vi "New_camera_Configuration_testcode.vi"(5 "Exposure time":dbl, 7 "Framerate":dbl, 8 "error in (no error)":errorcluster, 9 "CAM Model":enum16{"a2A5328-15ucBAS", "acA1920-155uc"}(ring), 10 "Camera":T2, 11 "Refnum in":T1) -> (0 "error out 2":errorcluster, 3 "Refnum out 2":T1)   [LabVIEW 2024]
uses:
  Camera_ID.ctl
  <vilib>/userDefined/High Color/IMAQdx.ctl
  <resource>/objmgr/imaqdx.rc
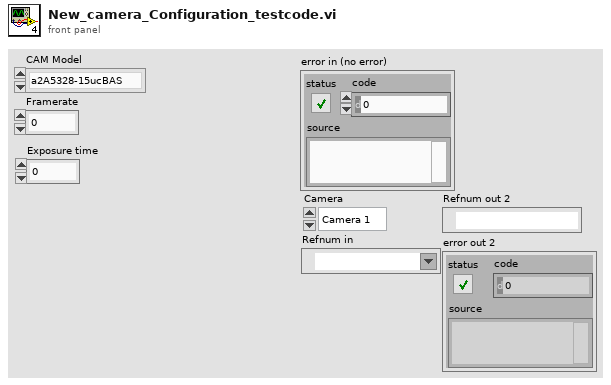
[diagram p1: front panel]
types:
  T1 = typedef "IMAQdx.ctl" = refnum<k21>
  T2 = typedef "Camera_ID.ctl" = enum16{"Camera 1", "Camera 2"}
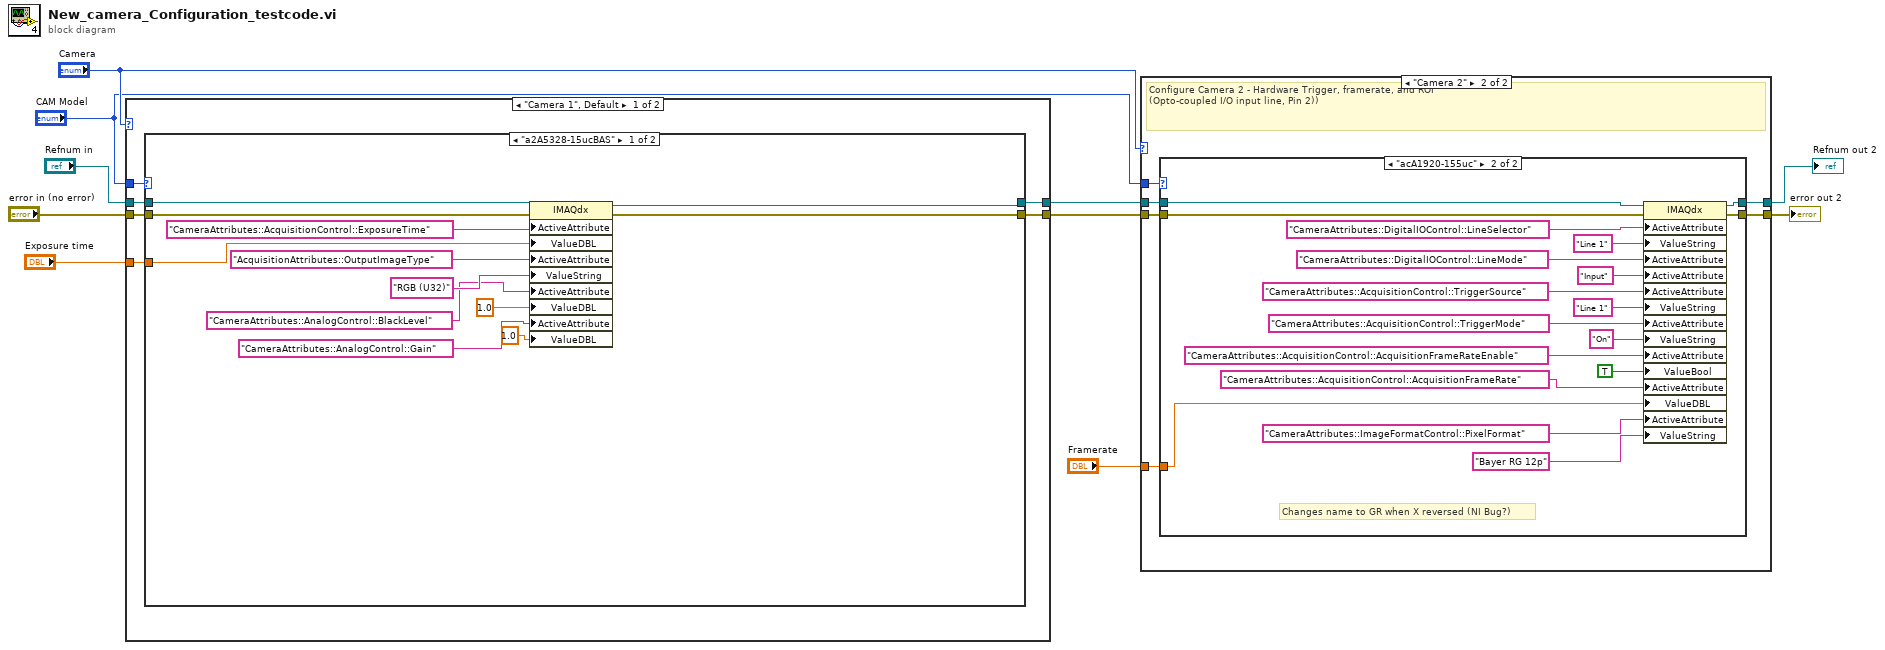
[diagram p0: block diagram]
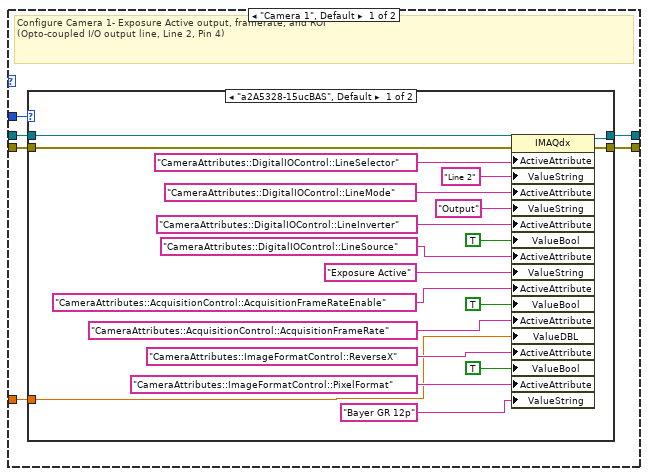
[diagram p2: hidden frame]
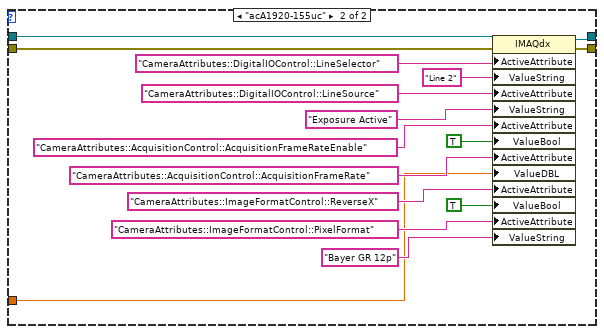
[diagram p3: hidden frame]
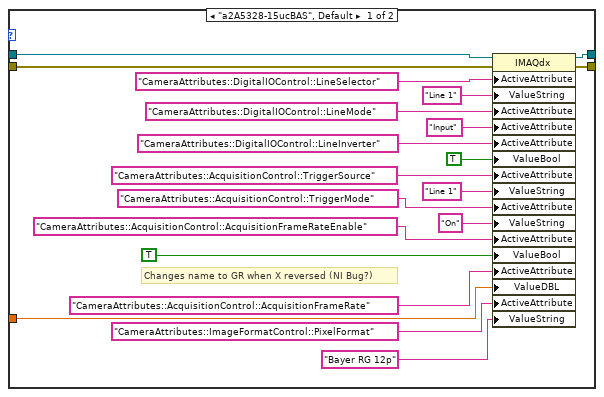
[diagram p4: hidden frame]
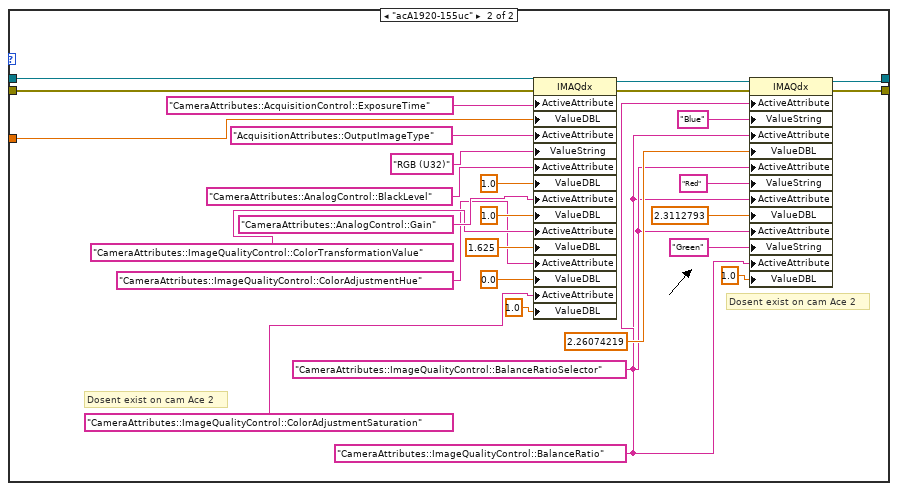
[diagram p5: hidden frame]
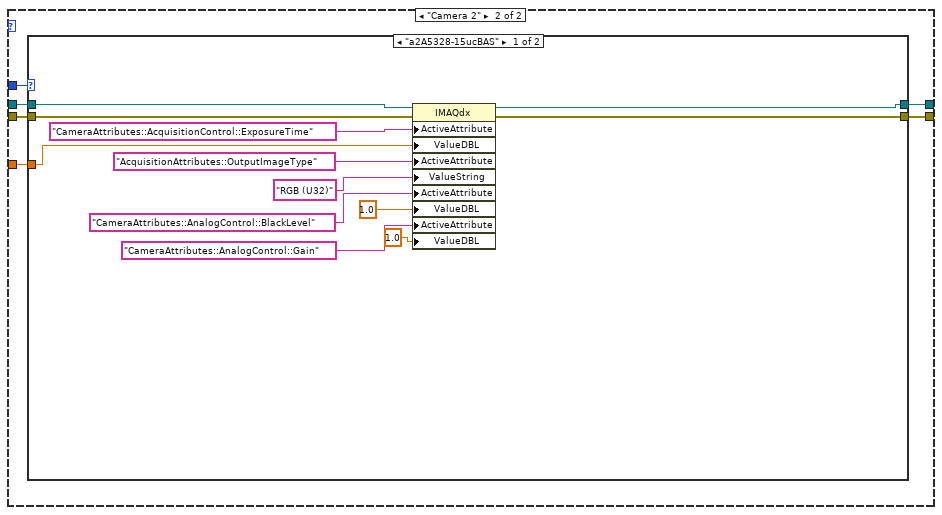
[diagram p6: hidden frame]
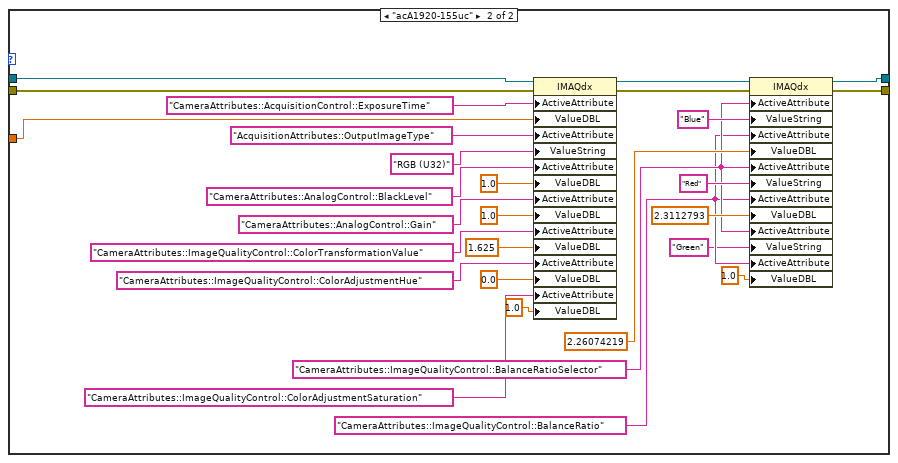
[diagram p7: hidden frame]
diagram:
  n1 = case shown="\"Camera 1\", Default" "Camera" {
    tunnel: "error in (no error)" -> [w15 w62]
    tunnel: [w16 w61] -> w7
    tunnel: "Refnum in" -> [w13 w60]
    tunnel: [w14 w59] -> w8
    tunnel: "CAM Model" -> [w12 w57]
    tunnel: "Exposure time" -> [w11 w58]
    frame "Camera 1", Default {
      n2 = case shown="\"a2A5328-15ucBAS\"" w12 {
        tunnel: w15 -> [w28 w33]
        tunnel: [w26 w32] -> w16
        tunnel: [w25 w31] -> w14
        tunnel: w13 -> [w27 w30]
        tunnel: w11 -> [w17 w29]
        frame "a2A5328-15ucBAS" {
          n3 = property class="IMAQdx"(reference=w27, error in=w28, "ActiveAttribute"="CameraAttributes::AcquisitionControl::ExposureTime", "ValueDBL"=w17, "ActiveAttribute"="AcquisitionAttributes::OutputImageType", "ValueString"="RGB (U32)", "ActiveAttribute"="CameraAttributes::AnalogControl::BlackLevel", "ValueDBL"=1.0, "ActiveAttribute"="CameraAttributes::AnalogControl::Gain", "ValueDBL"=1.0) -> (reference out=w25:T1, error out=w26:errorcluster)
        }
        frame "acA1920-155uc" {
          w38 = "CameraAttributes::ImageQualityControl::BalanceRatio" ("ActiveAttribute")
          w39 = "CameraAttributes::ImageQualityControl::BalanceRatioSelector" ("ActiveAttribute")
          # "Dosent exist on cam Ace 2"
          # "Dosent exist on cam Ace 2"
          n4 = property class="IMAQdx"(reference=w30, error in=w33, "ActiveAttribute"="CameraAttributes::AcquisitionControl::ExposureTime", "ValueDBL"=w29, "ActiveAttribute"="AcquisitionAttributes::OutputImageType", "ValueString"="RGB (U32)", "ActiveAttribute"="CameraAttributes::AnalogControl::BlackLevel", "ValueDBL"=1.0, "ActiveAttribute"="CameraAttributes::AnalogControl::Gain", "ValueDBL"=1.0, "ActiveAttribute"="CameraAttributes::ImageQualityControl::ColorTransformationValue", "ValueDBL"=1.625, "ActiveAttribute"="CameraAttributes::ImageQualityControl::ColorAdjustmentHue", "ValueDBL"=0.0, "ActiveAttribute"="CameraAttributes::ImageQualityControl::ColorAdjustmentSaturation", "ValueDBL"=1.0) -> (reference out=w55:T1, error out=w54:errorcluster)
          n5 = property class="IMAQdx"(reference=w55, error in=w54, "ActiveAttribute"=w39, "ValueString"="Blue", "ActiveAttribute"=w38, "ValueDBL"=2.26074219, "ActiveAttribute"=w39, "ValueString"="Red", "ActiveAttribute"=w38, "ValueDBL"=2.3112793, "ActiveAttribute"=w39, "ValueString"="Green", "ActiveAttribute"=w38, "ValueDBL"=1.0) -> (reference out=w31:T1, error out=w32:errorcluster)
        }
      }
    }
    frame "Camera 2" {
      n6 = case shown="\"a2A5328-15ucBAS\"" w57 {
        tunnel: w62 -> [w67 w79]
        tunnel: [w65 w78] -> w61
        tunnel: w60 -> [w66 w76]
        tunnel: [w64 w77] -> w59
        tunnel: w58 -> [w63 w75]
        frame "a2A5328-15ucBAS" {
          n7 = property class="IMAQdx"(reference=w66, error in=w67, "ActiveAttribute"="CameraAttributes::AcquisitionControl::ExposureTime", "ValueDBL"=w63, "ActiveAttribute"="AcquisitionAttributes::OutputImageType", "ValueString"="RGB (U32)", "ActiveAttribute"="CameraAttributes::AnalogControl::BlackLevel", "ValueDBL"=1.0, "ActiveAttribute"="CameraAttributes::AnalogControl::Gain", "ValueDBL"=1.0) -> (reference out=w64:T1, error out=w65:errorcluster)
        }
        frame "acA1920-155uc" {
          w84 = "CameraAttributes::ImageQualityControl::BalanceRatio" ("ActiveAttribute")
          w85 = "CameraAttributes::ImageQualityControl::BalanceRatioSelector" ("ActiveAttribute")
          n8 = property class="IMAQdx"(reference=w76, error in=w79, "ActiveAttribute"="CameraAttributes::AcquisitionControl::ExposureTime", "ValueDBL"=w75, "ActiveAttribute"="AcquisitionAttributes::OutputImageType", "ValueString"="RGB (U32)", "ActiveAttribute"="CameraAttributes::AnalogControl::BlackLevel", "ValueDBL"=1.0, "ActiveAttribute"="CameraAttributes::AnalogControl::Gain", "ValueDBL"=1.0, "ActiveAttribute"="CameraAttributes::ImageQualityControl::ColorTransformationValue", "ValueDBL"=1.625, "ActiveAttribute"="CameraAttributes::ImageQualityControl::ColorAdjustmentHue", "ValueDBL"=0.0, "ActiveAttribute"="CameraAttributes::ImageQualityControl::ColorAdjustmentSaturation", "ValueDBL"=1.0) -> (reference out=w101:T1, error out=w100:errorcluster)
          n9 = property class="IMAQdx"(reference=w101, error in=w100, "ActiveAttribute"=w85, "ValueString"="Blue", "ActiveAttribute"=w84, "ValueDBL"=2.26074219, "ActiveAttribute"=w85, "ValueString"="Red", "ActiveAttribute"=w84, "ValueDBL"=2.3112793, "ActiveAttribute"=w85, "ValueString"="Green", "ActiveAttribute"=w84, "ValueDBL"=1.0) -> (reference out=w77:T1, error out=w78:errorcluster)
        }
      }
    }
  }
  n10 = case shown="\"Camera 2\"" "Camera" {
    tunnel: w8 -> [w108 w150]
    tunnel: [w107 w149] -> w4
    tunnel: [w106 w148] -> w3
    tunnel: w7 -> [w105 w147]
    tunnel: "CAM Model" -> [w104 w146]
    tunnel: "Framerate" -> [w103 w145]
    frame "Camera 1", Default {
      # "Configure Camera 1- Exposure Active output, framerate, and ROI\n(Opto-coupled I/O output line, Line 2, Pin 4)"
      n11 = case shown="\"a2A5328-15ucBAS\", Default" w104 {
        tunnel: w108 -> [w128 w144]
        tunnel: [w126 w143] -> w107
        tunnel: [w125 w142] -> w106
        tunnel: w105 -> [w127 w140]
        tunnel: w103 -> [w109 w129]
        frame "a2A5328-15ucBAS", Default {
          n12 = property class="IMAQdx"(reference=w128, error in=w127, "ActiveAttribute"="CameraAttributes::DigitalIOControl::LineSelector", "ValueString"="Line 2", "ActiveAttribute"="CameraAttributes::DigitalIOControl::LineMode", "ValueString"="Output", "ActiveAttribute"="CameraAttributes::DigitalIOControl::LineInverter", "ValueBool"=TRUE, "ActiveAttribute"="CameraAttributes::DigitalIOControl::LineSource", "ValueString"="Exposure Active", "ActiveAttribute"="CameraAttributes::AcquisitionControl::AcquisitionFrameRateEnable", "ValueBool"=TRUE, "ActiveAttribute"="CameraAttributes::AcquisitionControl::AcquisitionFrameRate", "ValueDBL"=w109, "ActiveAttribute"="CameraAttributes::ImageFormatControl::ReverseX", "ValueBool"=TRUE, "ActiveAttribute"="CameraAttributes::ImageFormatControl::PixelFormat", "ValueString"="Bayer GR 12p") -> (reference out=w126:T1, error out=w125:errorcluster)
        }
        frame "acA1920-155uc" {
          n13 = property class="IMAQdx"(reference=w144, error in=w140, "ActiveAttribute"="CameraAttributes::DigitalIOControl::LineSelector", "ValueString"="Line 2", "ActiveAttribute"="CameraAttributes::DigitalIOControl::LineSource", "ValueString"="Exposure Active", "ActiveAttribute"="CameraAttributes::AcquisitionControl::AcquisitionFrameRateEnable", "ValueBool"=TRUE, "ActiveAttribute"="CameraAttributes::AcquisitionControl::AcquisitionFrameRate", "ValueDBL"=w129, "ActiveAttribute"="CameraAttributes::ImageFormatControl::ReverseX", "ValueBool"=TRUE, "ActiveAttribute"="CameraAttributes::ImageFormatControl::PixelFormat", "ValueString"="Bayer GR 12p") -> (reference out=w143:T1, error out=w142:errorcluster)
        }
      }
    }
    frame "Camera 2" {
      # "Configure Camera 2 - Hardware Trigger, framerate, and ROI \n(Opto-coupled I/O input line, Pin 2))"
      n14 = case shown="\"acA1920-155uc\"" w146 {
        tunnel: w150 -> [w155 w187]
        tunnel: [w157 w186] -> w149
        tunnel: [w156 w185] -> w148
        tunnel: w147 -> [w154 w184]
        tunnel: w145 -> [w151 w171]
        frame "a2A5328-15ucBAS", Default {
          # "Changes name to GR when X reversed (NI Bug?)"
          n15 = property class="IMAQdx"(reference=w155, error in=w154, "ActiveAttribute"="CameraAttributes::DigitalIOControl::LineSelector", "ValueString"="Line 1", "ActiveAttribute"="CameraAttributes::DigitalIOControl::LineMode", "ActiveAttribute"="Input", "ActiveAttribute"="CameraAttributes::DigitalIOControl::LineInverter", "ValueBool"=TRUE, "ActiveAttribute"="CameraAttributes::AcquisitionControl::TriggerSource", "ValueString"="Line 1", "ActiveAttribute"="CameraAttributes::AcquisitionControl::TriggerMode", "ValueString"="On", "ActiveAttribute"="CameraAttributes::AcquisitionControl::AcquisitionFrameRateEnable", "ValueBool"=TRUE, "ActiveAttribute"="CameraAttributes::AcquisitionControl::AcquisitionFrameRate", "ValueDBL"=w151, "ActiveAttribute"="CameraAttributes::ImageFormatControl::PixelFormat", "ValueString"="Bayer RG 12p") -> (reference out=w157:T1, error out=w156:errorcluster)
        }
        frame "acA1920-155uc" {
          # "Changes name to GR when X reversed (NI Bug?)"
          n16 = property class="IMAQdx"(reference=w187, error in=w184, "ActiveAttribute"="CameraAttributes::DigitalIOControl::LineSelector", "ValueString"="Line 1", "ActiveAttribute"="CameraAttributes::DigitalIOControl::LineMode", "ActiveAttribute"="Input", "ActiveAttribute"="CameraAttributes::AcquisitionControl::TriggerSource", "ValueString"="Line 1", "ActiveAttribute"="CameraAttributes::AcquisitionControl::TriggerMode", "ValueString"="On", "ActiveAttribute"="CameraAttributes::AcquisitionControl::AcquisitionFrameRateEnable", "ValueBool"=TRUE, "ActiveAttribute"="CameraAttributes::AcquisitionControl::AcquisitionFrameRate", "ValueDBL"=w171, "ActiveAttribute"="CameraAttributes::ImageFormatControl::PixelFormat", "ValueString"="Bayer RG 12p") -> (reference out=w186:T1, error out=w185:errorcluster)
        }
      }
    }
  }
  "Refnum out 2" <- w4
  "error out 2" <- w3
